vi "Read TrayStatus.vi"(8 "error in (no error)":errorcluster, 10 "F1/T2":bool, 11 "LineScan in":refnum<class "LineScan.lvclass">) -> (0 "error out":errorcluster, 1 "Arr_TrayST":bool[][](array[boolean]), 2 "Arr_Tray":cluster{"X":sgl, "Y":sgl}[][](array[cluster]), 3 "LineScan out":refnum<class "LineScan.lvclass">)   [LabVIEW 2019, in "LineScan.lvclass"]
uses:
  LineScan.lvclass
  Function/TraySet Folder/global/Tray_ArrAndData.vi
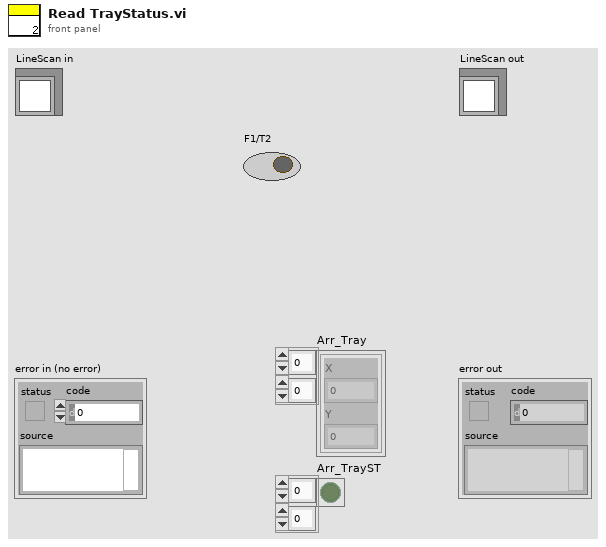
[diagram p1: front panel]
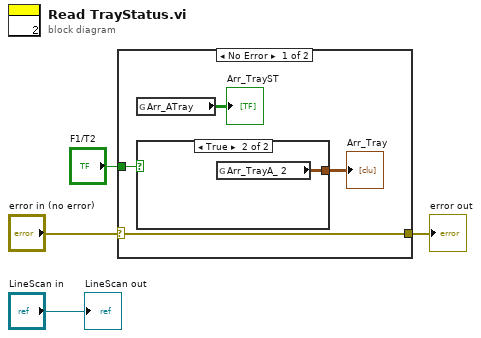
[diagram p0: block diagram]
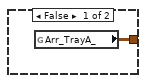
[diagram p2: hidden frame]
diagram:
  n1 = case shown="No Error" "error in (no error)" {
    selector: "error in (no error)" -> [w5 w11]
    tunnel: "F1/T2" -> [w6 _]
    tunnel: [w5 w11] -> w1
    frame No Error {
      n2 = global read "Tray_ArrAndData.vi" "Arr_ATray"() -> (→"Arr_TrayST":bool[][])
      n3 = case shown="True" w6 {
        tunnel: [w9 w10] -> w7
        frame False {
          n4 = global read "Tray_ArrAndData.vi" "Arr_TrayA_"() -> (w9:cluster{"X":sgl, "Y":sgl}[][])
        }
        frame True {
          n5 = global read "Tray_ArrAndData.vi" "Arr_TrayA_ 2"() -> (w10:cluster{"X":sgl, "Y":sgl}[][])
        }
      }
      "Arr_Tray" <- w7
    }
    frame Error {
    }
  }
  "error out" <- w1
  "LineScan out" <- "LineScan in"
